vi "Stepper Configure.vi"(6 "Control Method":u8(ring)=1 items=["2 Wire (Pulse & Direction)"=1, "2 Wire"=2, "4 Wire"=4, "EasyDriver"=6, "AF Motor Shield (Stepper 1 & 2 Only)"=5], 7 "Stepper #":u8, 8 "error in":errorcluster, 10 "Stepper Pins":u8[](array[numeric])=[2, 3], 11 "Arduino Resource":T1={"VISA resource"="", "Board Type"=enum."Uno", "Connection Type"=enum."USB / Serial", "Bytes Per Packet (15)"=15}) -> (0 "error out":errorcluster, 3 "Arduino Resource Out":T1={"VISA resource"="", "Board Type"=enum."Uno", "Connection Type"=enum."USB / Serial", "Bytes Per Packet (15)"=15})   [LabVIEW 2015, in "LabVIEW Interface for Arduino.lvlib"]
doc: "Specify a stepper #(0-7) and the digital pins for H-bridge based or step & direction stepper drivers. Specify a stepper #(0-1) without pins for use with the Adafruit Motor Shield."
uses:
  <vilib>/LabVIEW Interface for Arduino/LabVIEW Interface for Arduino.lvlib
  <vilib>/LabVIEW Interface for Arduino/Type Defs/Arduino Resource.ctl
  <vilib>/LabVIEW Interface for Arduino/Type Defs/Board Type.ctl
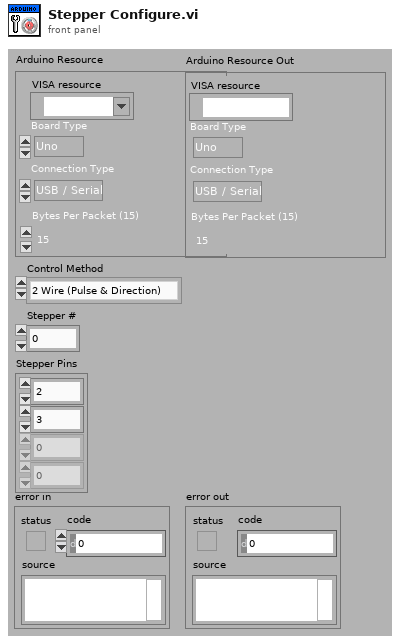
[diagram p1: front panel]
types:
  T1 = typedef "LabVIEW Interface for Arduino.lvlib/Arduino Resource.ctl" = cluster{"VISA resource":refnum<visa-resource-name>, "Board Type":T2, "Connection Type":enum8{"USB / Serial"}, "Bytes Per Packet (15)":u8}
  T2 = typedef "LabVIEW Interface for Arduino.lvlib/Board Type.ctl" = enum16{"Uno", "Dimuelanove w/Atmega 328", "Mega 2560"}
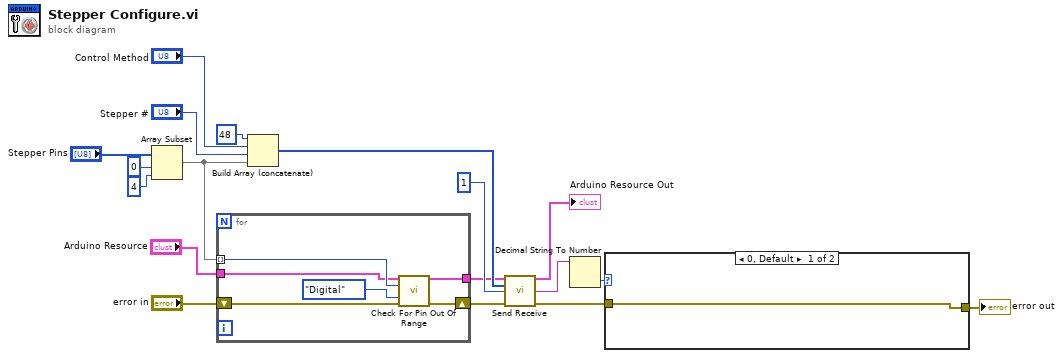
[diagram p0: block diagram]
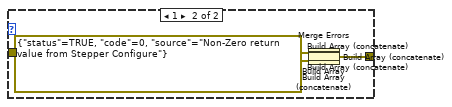
[diagram p2: hidden frame]
diagram:
  n1 = Array Subset(array="Stepper Pins", index=0, length=4) -> (w5:u8[])
  n2 = for {
    tunnel: w5 -> [w24] mode=indexing
    tunnel: "Arduino Resource" -> [w22]
    tunnel: [w21] -> w8
    shift-right: [w19] -> w9
    shift-left: "error in" -> [w20]
    n3 = call <vilib>:"Check For Pin Out Of Range.vi"("Arduino Resource"=w22, "User Pin Number"=w24, "Pin Type"=enum16{"Analog", "Digital"}."Digital", "error in"=w20) -> ("Arduino Resource"=w21:T1, "error out"=w19:errorcluster)  [unwired: 10 in]
  }
  n4 = Build Array (concatenate)(u8 48, "Control Method", "Stepper #", w5) -> (w14:u8[])
  n5 = call <vilib>:"Send Receive.vi"("Arduino Resource"=w8, "Data"=w14, "Bytes To Read (0)"=u8 1, "error in"=w9) -> ("Arduino Resource"=→"Arduino Resource Out":T1, "Read Buffer"=w1:string, "error out"=w4:errorcluster)  [unwired: 9 in]
  n6 = Decimal String To Number(string=w1) -> (number=w2:i32)  [unwired: 2 in, 1 out]
  n7 = case shown="0, Default" w2 {
    tunnel: w4 -> [w25 w33]
    tunnel: [w25 w32] -> w3
    frame 0, Default {
    }
    frame 1 {
      n8 = Build Array(w33, errorcluster {"status"=TRUE, "code"=0, "source"="Non-Zero return value from Stepper Configure"} ("error in")) -> (w30:errorcluster[])
      n9 = Build Array (concatenate)(w30) -> (w29:errorcluster[])
      n10 = Build Array (concatenate)(w29) -> (w28:errorcluster[])
      n11 = Build Array (concatenate)(w28) -> (w27:errorcluster[])
      n12 = Build Array (concatenate)(w27) -> (w26:errorcluster[])
      n13 = Merge Errors(w26) -> (w32:errorcluster)
    }
  }
  "error out" <- w3
